vi "PV MiniTest Operating.vi"(8 "error in (no error)":errorcluster, 9 "Operating adjustment - Cluster":T1 {"Pressure gauge upper\nrange value" items=[" 0,1 mbar", " 1 mbar", " 10 mbar", " 100 mbar", " 1000 mbar", " 2000 mbar", " 5000 mbar", " 10000 mbar", " 50000 mbar"]; "Parameter" items=[" Pressure gauge upper range value", " Software version MiniTest 300 (read only)", " Operating hours [h] (read only)", " Device name (read only)", " MiniTest serial number (read only)"]}, 10 "Adress of unit":u16=1 min=1 max=999 step=1, 11 "VISA session":refnum<visa-resource-name>) -> (0 "error out":errorcluster, 2 "response (data)":string, 3 "dup VISA session":refnum<visa-resource-name>)   [LabVIEW 2021, in "Pfeiffer Vacuum.lvlib"]
doc: "There are 5 parameters available, only one of which can be enabled at a time. \n\n0 - Pressure gauge upper range value (default) Para. 16\n1 - Software version MiniTest 300 (read only) Para. 312\n2 - Operating hours [h] (read only) Para. 314\n3 - Device name (read only) Para. 349\n4 - MiniTest serial number (read only) Para. 355\n\nNote: The one control right of this one will set the appropriate values for the selected parameter. Any settings for an parameter that is not selected will be ignored. If a value is out of range, it will be changed to either the upper or the lower limit of the range."
uses:
  <instrlib>/Pfeiffer Vacuum/Pfeiffer Vacuum.lvlib
  <instrlib>/Pfeiffer Vacuum/Public/MiniTest/PV MiniTest Operating - Cluster.ctl
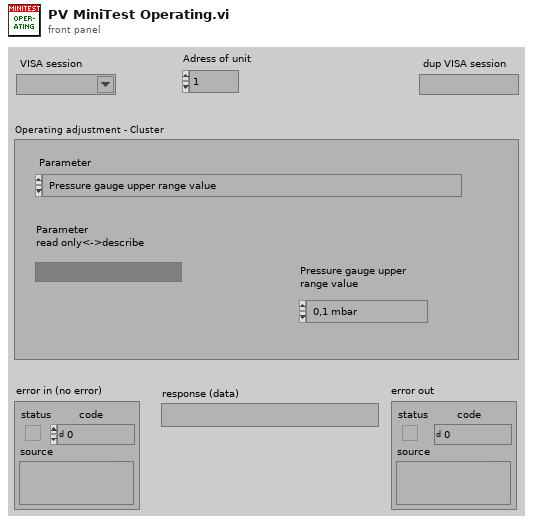
[diagram p1: front panel]
types:
  T1 = typedef "Pfeiffer Vacuum.lvlib/PV MiniTest Operating - Cluster.ctl" = cluster{"Parameter":u16, "Parameter\nread only<->describe":bool, "Pressure gauge upper\nrange value":u16}
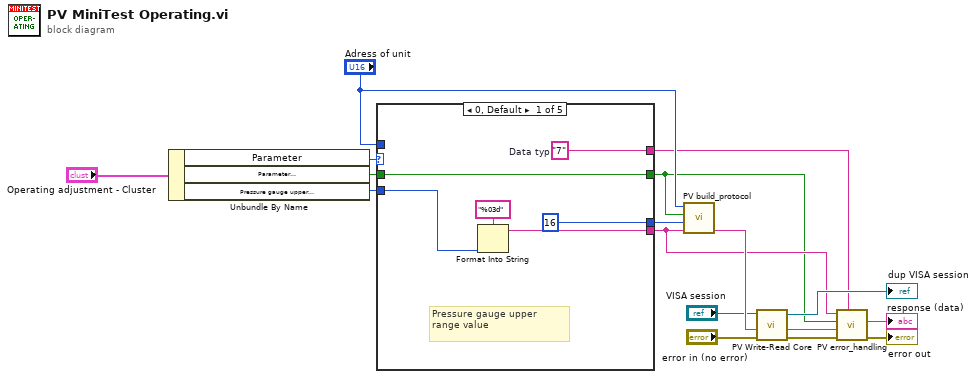
[diagram p0: block diagram]
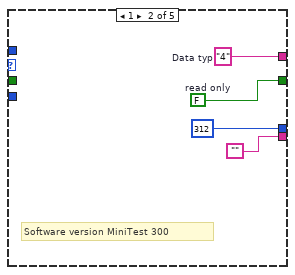
[diagram p2: hidden frame]
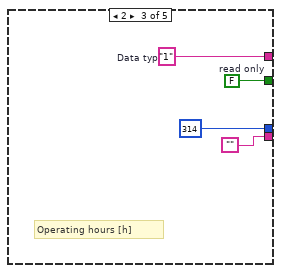
[diagram p3: hidden frame]
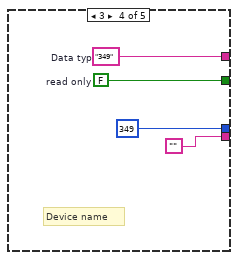
[diagram p4: hidden frame]
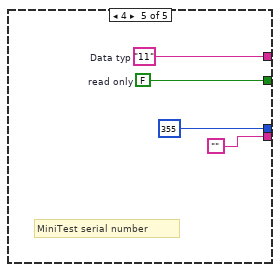
[diagram p5: hidden frame]
diagram:
  n1 = Unbundle By Name("Operating adjustment - Cluster") -> ("Parameter"=w1:u16, "Parameter\nread only<->describe"=w15:bool, "Pressure gauge upper\nrange value"=w2:u16)
  n2 = case shown="0, Default" w1 {
    tunnel: [u16 16 ("Parameter-number") u16 312 ("Parameter-number") u16 314 ("Parameter-number") u16 349 ("Parameter-number") u16 355 ("Parameter-number")] -> w17
    tunnel: [w19 "" "" "" ""] -> w9
    tunnel: [w21 w26 w28 w34 w38] -> w7
    tunnel: w15 -> [w21 _ _ _ _]
    tunnel: [w22 w27 w31 w35 w39] -> w8
    tunnel: "Adress of unit" -> [_ _ _ _ _]
    tunnel: w2 -> [w18 _ _ _ _]
    frame 0, Default {
      w22 = "7"  # Data typ
      # "Pressure gauge upper\nrange value"
      n3 = Format Into String(format string="%03d" ("Format-String"), w18) -> (resulting string=w19:string)  [unwired: 2 in, 1 out]
    }
    frame 1 {
      w27 = "4"  # Data typ
      w26 = FALSE  # read only
      # "Software version MiniTest 300"
    }
    frame 2 {
      w28 = FALSE  # read only
      w31 = "1"  # Data typ
      # "Operating hours [h]"
    }
    frame 3 {
      w35 = "349"  # Data typ
      w34 = FALSE  # read only
      # "Device name"
    }
    frame 4 {
      w39 = "11"  # Data typ
      w38 = FALSE  # read only
      # "MiniTest serial number"
    }
  }
  n4 = call <instrlib>:"PV build_protocol.vi"("Data"=w9, "Parameter-number"=w17, "parameter\nread<->describe"=w7, "Adress"="Adress of unit") -> ("output"=w13:string)  [unwired: 3 in]
  n5 = call <instrlib>:"PV Write-Read Core.vi"("error in"="error in (no error)", "Write data in"=w13, "VISA session"="VISA session") -> ("error out"=w11:errorcluster, "response (data) out"=w12:string, "dup VISA session"=→"dup VISA session":refnum<visa-resource-name>)  [unwired: 2 in]
  n6 = call <instrlib>:"PV error_handling.vi"("Data Typ in"=w8, "error in"=w11, "response (data) in"=w12, "Parameter\nread only<->describe"=w7, "data in"=w9) -> ("error out"=→"error out":errorcluster, "Data out"=→"response (data)":string)  [unwired: 4 in, 1 out]
